vi "Configure SMU.vi"(5 "aperture time":dbl=0.001, 7 "Source Mode":enum16{"Voltage", "Current"}(ring), 8 "error in (no error)":errorcluster, 9 "Settings":T2 {"Sense" items=["Local"=1008, "Remote"=1009]}, 10 "Pins":string[](array[string]), 11 "Semiconductor Module Context":T3) -> (0 "error out":errorcluster)   [LabVIEW 2013]
uses:
  <vilib>/NI_TestStand_SemiconductorModule/NI_TestStand_Semiconductor_Module.lvlibp/PinMap/General/SemiconductorModuleContext.ctl
  <instrlib>/niDCPower/nidcpower.llb/niDCPower Sense.ctl
  <instrlib>/niDCPower/nidcpower.llb/niDCPower Aperture Time Units.ctl
  <instrlib>/niDCPower/nidcpower.llb/niDCPower Output Function.ctl
  <vilib>/NI_TestStand_SemiconductorModule/NI_TestStand_Semiconductor_Module.lvlibp/PinMap/DC Power/PinsToNIDCPowerSessions.vi
  <vilib>/NI_TestStand_SemiconductorModule/NI_TestStand_Semiconductor_Module.lvlibp
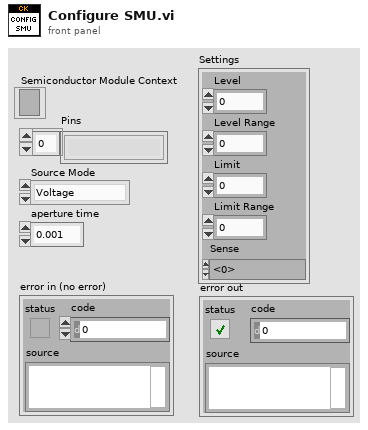
[diagram p1: front panel]
types:
  T1 = typedef "niDCPower Sense.ctl" = i32
  T2 = cluster{"Level":dbl, "Level Range":dbl, "Limit":dbl, "Limit Range":dbl, "Sense":T1}
  T3 = typedef "NI_TestStand_Semiconductor_Module.lvlibp/SemiconductorModuleContext.ctl" = refnum<k7>
  T4 = typedef "niDCPower Aperture Time Units.ctl" = i32
  T5 = typedef "niDCPower Output Function.ctl" = i32
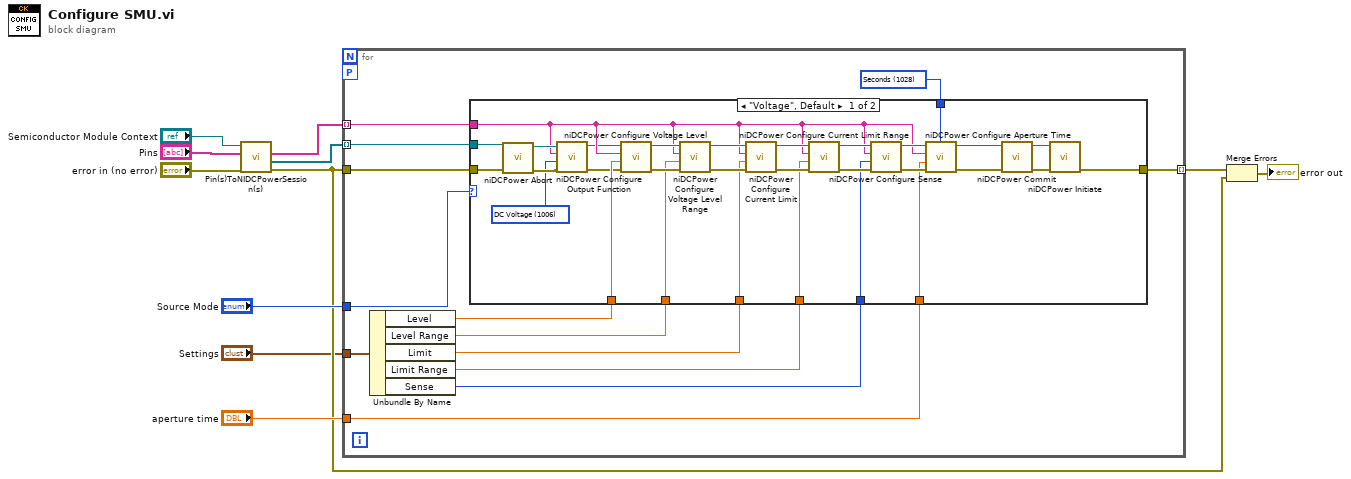
[diagram p0: block diagram]
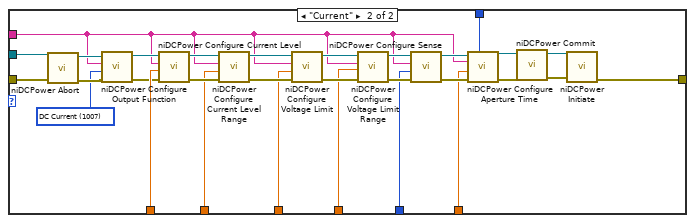
[diagram p2: hidden frame]
diagram:
  n1 = call-poly <vilib>:"Pin(s)ToNIDCPowerSession(s).vi"("error in (no error)"="error in (no error)", "Pins"="Pins", "Semiconductor Module Context"="Semiconductor Module Context") -> ("error out"=w3:errorcluster, "Instrument Sessions"=w9:refnum<k15>[], "Channel Lists"=w8:string[])  [unwired: 4 in, 2 out]
  n2 = for {
    tunnel: w9 -> [w23] mode=indexing
    tunnel: w8 -> [w22] mode=indexing
    tunnel: "Settings" -> [w20]
    tunnel: "Source Mode" -> [w15]
    tunnel: "aperture time" -> [w12]
    tunnel: w3 -> [w24]
    tunnel: [w21] -> w5 mode=indexing
    workers-P: _ -> [_]
    w13 = T4 1028 items=["Seconds"=1028, "Powerline Cycles"=1029] ("aperture time units")
    n3 = Unbundle By Name(w20) -> ("Level"=w19:dbl, "Level Range"=w18:dbl, "Limit"=w17:dbl, "Limit Range"=w16:dbl, "Sense"=w14:T1)
    n4 = case shown="\"Voltage\", Default" w15 {
      tunnel: w24 -> [w26 w66]
      tunnel: w23 -> [w28 w65]
      tunnel: w22 -> [w29 w60]
      tunnel: [w46 w74] -> w21
      tunnel: w19 -> [w45 w84]
      tunnel: w18 -> [w44 w81]
      tunnel: w17 -> [w43 w78]
      tunnel: w16 -> [w42 w75]
      tunnel: w14 -> [w37 w71]
      tunnel: w12 -> [w39 w68]
      tunnel: w13 -> [w38 w67]
      frame "Voltage", Default {
        w30 = T5 1006 items=["DC Voltage"=1006, "DC Current"=1007, "Pulse Voltage"=1049, "Pulse Current"=1050] ("output function")
        n5 = call <instrlib>:"niDCPower Abort.vi"("error in (no error)"=w26, "instrument handle"=w28) -> ("error out"=w32:errorcluster, "instrument handle out"=w31:refnum<k15>)  [unwired: 8 in]
        n6 = call <instrlib>:"niDCPower Configure Output Function.vi"("error in (no error)"=w32, "output function"=w30, "channel name"=w29, "instrument handle"=w31) -> ("error out"=w25:errorcluster, "instrument handle out"=w27:refnum<k15>)  [unwired: 6 in]
        n7 = call <instrlib>:"niDCPower Configure Voltage Level.vi"("error in (no error)"=w25, "voltage level"=w45, "channel name"=w29, "instrument handle"=w27) -> ("error out"=w54:errorcluster, "instrument handle out"=w53:refnum<k15>)  [unwired: 6 in]
        n8 = call <instrlib>:"niDCPower Configure Voltage Level Range.vi"("error in (no error)"=w54, "voltage level range"=w44, "channel name"=w29, "instrument handle"=w53) -> ("error out"=w52:errorcluster, "instrument handle out"=w50:refnum<k15>)  [unwired: 6 in]
        n9 = call <instrlib>:"niDCPower Configure Current Limit.vi"("error in (no error)"=w52, "current limit"=w43, "channel name"=w29, "instrument handle"=w50) -> ("error out"=w51:errorcluster, "instrument handle out"=w49:refnum<k15>)  [unwired: 6 in]
        n10 = call <instrlib>:"niDCPower Configure Current Limit Range.vi"("error in (no error)"=w51, "current limit range"=w42, "channel name"=w29, "instrument handle"=w49) -> ("error out"=w48:errorcluster, "instrument handle out"=w47:refnum<k15>)  [unwired: 6 in]
        n11 = call <instrlib>:"niDCPower Configure Sense.vi"("error in (no error)"=w48, "sense"=w37, "channel name"=w29, "instrument handle"=w47) -> ("error out"=w41:errorcluster, "instrument handle out"=w40:refnum<k15>)  [unwired: 6 in]
        n12 = call <instrlib>:"niDCPower Configure Aperture Time.vi"("aperture time units"=w38, "error in (no error)"=w41, "aperture time"=w39, "channel name"=w29, "instrument handle"=w40) -> ("error out"=w35:errorcluster, "instrument handle out"=w36:refnum<k15>)  [unwired: 5 in]
        n13 = call <instrlib>:"niDCPower Commit.vi"("error in (no error)"=w35, "instrument handle"=w36) -> ("error out"=w34:errorcluster, "instrument handle out"=w33:refnum<k15>)  [unwired: 8 in]
        n14 = call <instrlib>:"niDCPower Initiate.vi"("error in (no error)"=w34, "instrument handle"=w33) -> ("error out"=w46:errorcluster)  [unwired: 8 in, 1 out]
      }
      frame "Current" {
        w59 = T5 1007 items=["DC Voltage"=1006, "DC Current"=1007, "Pulse Voltage"=1049, "Pulse Current"=1050] ("output function")
        n15 = call <instrlib>:"niDCPower Abort.vi"("error in (no error)"=w66, "instrument handle"=w65) -> ("error out"=w62:errorcluster, "instrument handle out"=w61:refnum<k15>)  [unwired: 8 in]
        n16 = call <instrlib>:"niDCPower Configure Output Function.vi"("error in (no error)"=w62, "output function"=w59, "channel name"=w60, "instrument handle"=w61) -> ("error out"=w64:errorcluster, "instrument handle out"=w63:refnum<k15>)  [unwired: 6 in]
        n17 = call <instrlib>:"niDCPower Configure Current Level.vi"("error in (no error)"=w64, "current level"=w84, "channel name"=w60, "instrument handle"=w63) -> ("error out"=w83:errorcluster, "instrument handle out"=w82:refnum<k15>)  [unwired: 6 in]
        n18 = call <instrlib>:"niDCPower Configure Current Level Range.vi"("error in (no error)"=w83, "current level range"=w81, "channel name"=w60, "instrument handle"=w82) -> ("error out"=w80:errorcluster, "instrument handle out"=w79:refnum<k15>)  [unwired: 6 in]
        n19 = call <instrlib>:"niDCPower Configure Voltage Limit.vi"("error in (no error)"=w80, "voltage limit"=w78, "channel name"=w60, "instrument handle"=w79) -> ("error out"=w77:errorcluster, "instrument handle out"=w76:refnum<k15>)  [unwired: 6 in]
        n20 = call <instrlib>:"niDCPower Configure Voltage Limit Range.vi"("error in (no error)"=w77, "voltage limit range"=w75, "channel name"=w60, "instrument handle"=w76) -> ("error out"=w73:errorcluster, "instrument handle out"=w72:refnum<k15>)  [unwired: 6 in]
        n21 = call <instrlib>:"niDCPower Configure Sense.vi"("error in (no error)"=w73, "sense"=w71, "channel name"=w60, "instrument handle"=w72) -> ("error out"=w70:errorcluster, "instrument handle out"=w69:refnum<k15>)  [unwired: 6 in]
        n22 = call <instrlib>:"niDCPower Configure Aperture Time.vi"("aperture time units"=w67, "error in (no error)"=w70, "aperture time"=w68, "channel name"=w60, "instrument handle"=w69) -> ("error out"=w56:errorcluster, "instrument handle out"=w55:refnum<k15>)  [unwired: 5 in]
        n23 = call <instrlib>:"niDCPower Commit.vi"("error in (no error)"=w56, "instrument handle"=w55) -> ("error out"=w57:errorcluster, "instrument handle out"=w58:refnum<k15>)  [unwired: 8 in]
        n24 = call <instrlib>:"niDCPower Initiate.vi"("error in (no error)"=w57, "instrument handle"=w58) -> ("error out"=w74:errorcluster)  [unwired: 8 in, 1 out]
      }
    }
  }
  n25 = Merge Errors(w5, w3) -> (→"error out":errorcluster)
